vi "DSF.Engine.Memory.Cache.Transfer.Get VS Channels Pointer.vi"(8 "error in (no error)":errorcluster, 11 "Transfer Cache in":refnum<class "DSF.Engine.Memory.Cache.Transfer.lvclass">) -> (0 "error out":errorcluster, 2 "VS Channels Pointer":refnum<class "DSF.Engine.Memory.Pointer.VS Channels.lvclass">, 3 "Transfer Cache out":refnum<class "DSF.Engine.Memory.Cache.Transfer.lvclass">)   [LabVIEW 2016, in "DSF.Engine.lvlib" / "DSF.Engine.Memory.Cache.Transfer.lvclass"]
uses:
  DSF.Engine.Memory.Cache.Transfer.lvclass
  Memory.Pointer/DSF.Engine.Memory.Pointer.VS Channels.lvclass
  DSF.Engine.Memory.Cache.Transfer.lvclass/DSF.Engine.Memory.Cache.Transfer.ctl
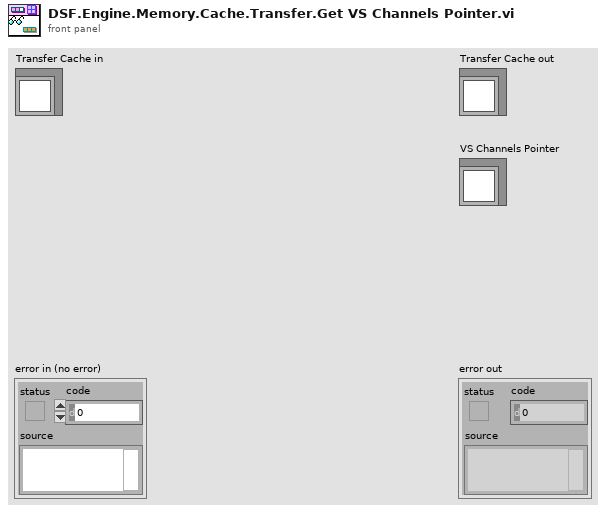
[diagram p1: front panel]
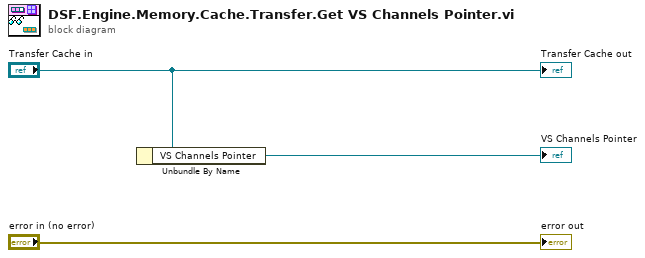
[diagram p0: block diagram]
diagram:
  n1 = Unbundle By Name("Transfer Cache in") -> ("VS Channels Pointer"=→"VS Channels Pointer":refnum<class "DSF.Engine.Memory.Pointer.VS Channels.lvclass">)
  "error out" <- "error in (no error)"
  "Transfer Cache out" <- "Transfer Cache in"
